vi "VsEP-Plot Traces.vi"(0 "Analysis":T2, 7 "Graphs":T1, 11 "error in":errorcluster, 12 "Normalize individual?":bool) -> (15 "error out":errorcluster)   [LabVIEW 2020]
uses:
  Typedefs/VsEP-Analysis State.ctl
  Typedefs/VsEP-Graph Controls.ctl
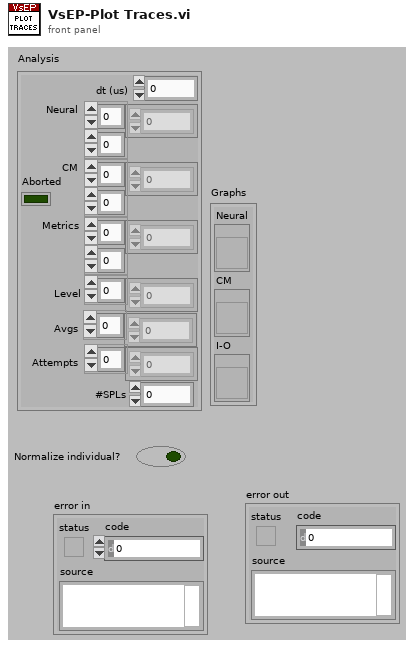
[diagram p1: front panel]
types:
  T1 = typedef "VsEP-Graph Controls.ctl" = cluster{"Neural":refnum<vi>, "CM":refnum<vi>, "I-O":refnum<vi>}
  T2 = typedef "VsEP-Analysis State.ctl" = cluster{"dt (us)":dbl, "Neural":dbl[][], "CM":dbl[][], "Metrics":dbl[][], "Level":dbl[], "Avgs":i32[], "Attempts":i32[], "Aborted":bool, "#SPLs":i32}
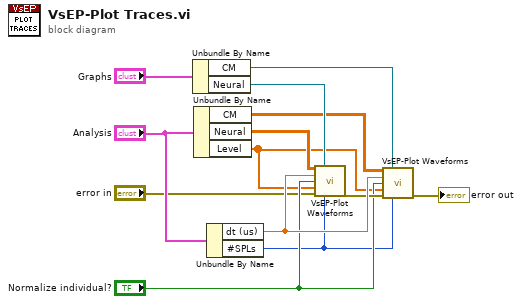
[diagram p0: block diagram]
diagram:
  n1 = Unbundle By Name("Graphs") -> ("CM"=w7:refnum<vi>, "Neural"=w11:refnum<vi>)
  n2 = Unbundle By Name("Analysis") -> ("CM"=w3:dbl[][], "Neural"=w4:dbl[][], "Level"=w1:dbl[])
  n3 = Unbundle By Name("Analysis") -> ("dt (us)"=w10:dbl, "#SPLs"=w6:i32)
  n4 = call "VsEP-Plot Waveforms.vi"("Array"=w4, "graph ref"=w11, "dt (us)"=w10, "Normalize traces"="Normalize individual?", "Sequence values"=w1, "error in (no error)"="error in", "Max #SPL"=w6) -> ("error out"=w9:errorcluster)  [unwired: 7 in, 1 out]
  n5 = call "VsEP-Plot Waveforms.vi"("Array"=w3, "graph ref"=w7, "dt (us)"=w10, "Normalize traces"="Normalize individual?", "Sequence values"=w1, "error in (no error)"=w9, "Max #SPL"=w6) -> ("error out"=→"error out":errorcluster)  [unwired: 7 in, 1 out]
